vi "rect.vi"() -> ()   [LabVIEW 2009]
uses:
  <vilib>/imath/engines/lvmath2/RunTimeEngine/ErrorHandling/NIMS_Finalize Error.vi
  <vilib>/imath/engines/lvmath2/RunTimeEngine/Parser/MC_Version.vi
  <vilib>/imath/engines/lvmath2/RunTimeEngine/NodeEndStatement/NIMS_NodeEndStatement_Output.vi
  <instcachedir>/0/NIMS_NodeEndStatement_Output_53EC0D466D134D7ABD903AC30B43404B.lvgen/NIMS_NodeEndStatement_Output_53EC0D466D134D7ABD903AC30B43404B_001.vi
  <vilib>/imath/engines/lvmath2/RunTimeEngine/RangeToken/NIMS_Range.vi
  <instcachedir>/0/NIMS_Range_08574DECC23E450FAF0AC0BC39E6BEA7.lvgen/NIMS_Range_08574DECC23E450FAF0AC0BC39E6BEA7_001.vi
  <vilib>/imath/engines/lvmath/Functions/Error Handling/MergeErrorsWrapper.vi
  <vilib>/imathl/engines/lvmath/Functions/Error Handling/Create Error.vi
  <vilib>/imath/engines/lvmath2/RunTimeEngine/BuiltInFunctions/zeros/NIMS_V=zeros(I32,I32).vi
  <vilib>/imath/engines/lvmath/Functions/Error Handling/MC_Error Cluster From Error Code.vi
  <vilib>/imath/engines/lvmath2/RunTimeEngine/BuiltInFunctions/fft/NIMS_fft(GV).vi
  <instcachedir>/0/NIMS_fft(GV)_4C6467FC22F84E4BA42517A07EF978B0.lvgen/NIMS_fft(GV)_4C6467FC22F84E4BA42517A07EF978B0_001.vi
  <vilib>/imath/engines/lvmath2/RunTimeEngine/BuiltInFunctions/abs/NIMS_abs(signed).vi
  <instcachedir>/0/NIMS_abs(signed)_C4FCB8E6058B49B797C7C8D53CA5F6EC.lvgen/NIMS_abs(signed)_C4FCB8E6058B49B797C7C8D53CA5F6EC_000.vi
  <vilib>/imath/engines/lvmath2/RunTimeEngine/BuiltInFunctions/fftshift/NIMS_fftshift(GV).vi
  <instcachedir>/0/NIMS_fftshift(GV)_BD7A7BA9CA6B470B9A9F73A6A3FEEB3E.lvgen/NIMS_fftshift(GV)_BD7A7BA9CA6B470B9A9F73A6A3FEEB3E_000.vi
panel:
  out "DFT":cluster{dbl[], dbl[]}(graph)
  out "Rectangular Pulse":cluster{dbl[], dbl[]}(graph)
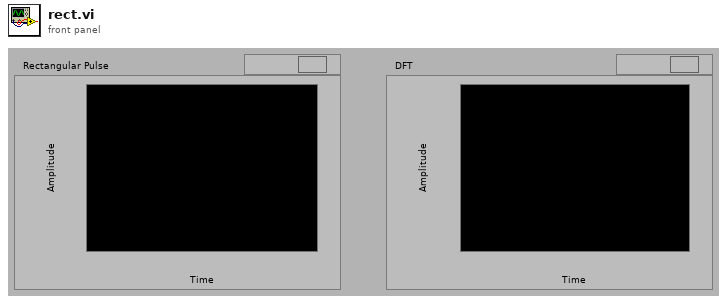
[diagram p1: front panel]
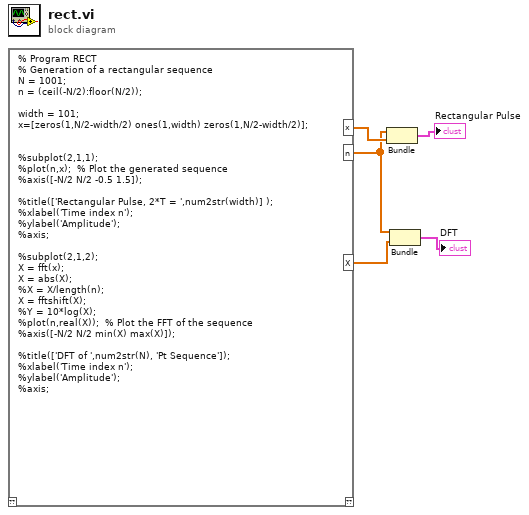
[diagram p0: block diagram]
diagram:
  n1 = mathscript code="% Program RECT\n% Generation of a rectangular sequence\nN = 1001;\nn = (ceil(-N/2):floor(N/2));\n\nwidth = 101;\nx=[zeros(1,N/2-width/2) ones(1,width) zeros(1,N/2-width/2)];\n\n\n%subplot(2,1,1);\n%plot(n,x);\t\t% Plot the generated sequence\n%axis([-N/2 N/2 -0.5 1.5]);\n\n%title(['Rectangular Pulse, 2*T = ',num2str(width)] );\n%xlabel('Time index n');\n%ylabel('Amplitude');\n%axis;\n\n%subplot(2,1,2);\nX = fft(x);\nX = abs(X);\n%X = X/length(n);\nX = fftshift(X);\n%Y = 10*log(X);\n%plot(n,real(X));\t\t% Plot the FFT of the sequence\n%axis([-N/2 N/2 min(X) max(X)]);\n \n%title(['DFT of ',num2str(N), 'Pt Sequence']);\n%xlabel('Time index n');\n%ylabel('Amplitude');\n%axis;"() -> ("x"=w5:dbl[], "X"=w2:dbl[], "n"=w3:dbl[])  [unwired: 1 in, 1 out]
  n2 = Bundle(w3, w5) -> (→"Rectangular Pulse":cluster{dbl[], dbl[]})  [unwired: 1 in]
  n3 = Bundle(w3, w2) -> (→"DFT":cluster{dbl[], dbl[]})  [unwired: 1 in]
